vi "Torque_2.vi"() -> ()   [LabVIEW 2020]
uses:
  Support/Controls/Cmd_Mouse Popup.ctl
  Support/Controls/Clst_Initialize Input.ctl
  Support/Controls/Cmd_Var Data IO.ctl
  Variables/Global_Cal Info.vi
  Variables/Global_Constant.vi
panel:
  in  "타입":string
  in  "Measured CCW_ADJ":string[][](table) caption="● 조정후 지시값 (반시계방향)"
  in  "Measured CW_ADJ":string[][](table) caption="● 조정후 지시값 (시계방향)"
  in  "Measured CCW":string[][](table) caption="● 토크 교정기 지시값 (반시계방향)"
  in  "측정방향":enum16{"양방향", "시계방향", "반시계방향"}(ring)
  in  "Spec 변경":bool
  in  "Random":bool
  out "Spec":string[][](table) caption="Spec (N·m)"
  out "제목":string
  out "에러 출력":errorcluster
  out "Condition":string[][](table) caption="○ 토크렌치 정확도 교정"
  in  "최소눈금":string(combo)
  out "단위":string
  out "최대용량":string
  in  "Measured CW":string[][](table) caption="● 토크 교정기 지시값 (시계방향)"
  out "Load?":bool
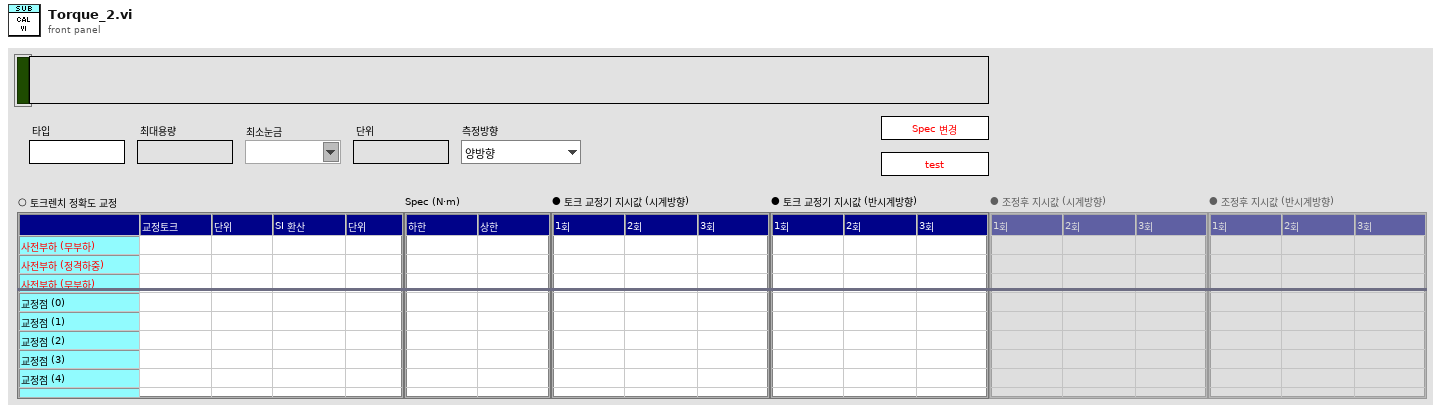
[diagram p1: front panel]
types:
  T1 = typedef "Clst_Cal Info Global.ctl" = cluster{"등록번호":string, "의뢰기관":string, "기기명":string, "제작회사":string, "형식":string, "기기번호":string, "소분류코드":string, "세부분류코드":string, "교정주기":string, "접수번호":string, "교정일자":string, "교정절차서 1":string, "교정절차서 2":string, "교정절차서 3":string, "접수확인자":string, "인증교정자":string, "기술책임자":string, "KOLAS 유무":string, "진행상태":string, "의뢰기관코드":string, "입고형태":string, "영문성적서?":bool, "합불판정?":bool, "부록?":bool, "절차서번호 1":string, "절차서번호 2":string, "절차서번호 3":string, "교정방식":string, "부서명":string}
  T2 = typedef "Cmd_Mouse Popup.ctl" = enum16{"활성화", "메뉴선택"}
  T3 = cluster{"Shift":bool, "Ctrl":bool, "Alt":bool, "Cmd":bool, "Opt":bool}
  T4 = typedef "Clst_Initialize Input.ctl" = cluster{"Initialize 1":cluster{"Condition":refnum<vi>[], "Spec":refnum<vi>[], "Measured":refnum<vi>[], "Resolution":refnum<vi>[], "Func_ext":string, "제목":refnum<vi>, "Measured_ADJ":refnum<vi>[]}, "Initialize 2":cluster{"문자열":refnum<vi>[], "콤보박스":refnum<vi>[], "링":refnum<vi>[], "열거형":refnum<vi>[], "테이블":refnum<vi>[], "여러열":refnum<vi>[], "디지털(DBL)":refnum<vi>[], "3D string":refnum<vi>[], "ctrl":refnum<vi>[], "boolean":refnum<vi>[]}}
  T5 = typedef "Cmd_Var Data IO.ctl" = enum16{"Condition", "Condition Default", "Condition_Temp", "Resolution", "Resolution Default", "Resolution Old", "Spec", "Spec Default", "Spec Old", "Spec Temp", "Result", "Result2", "Result3", "Result_Temp", "Result_ADJ", "Result_ADJ2", "STD1", "STD2", "STD3", "STD4", "STD5", "STD Temp", "CMC", "CMC Default"}
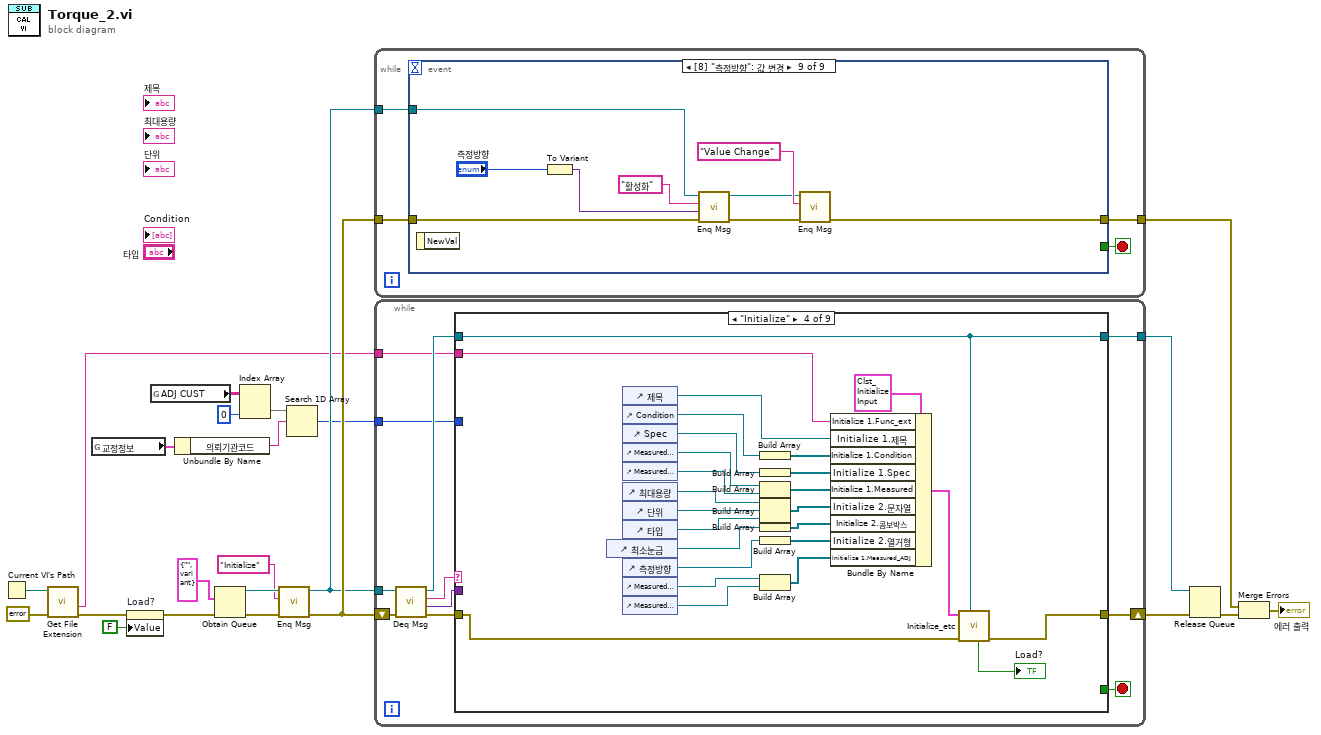
[diagram p0: block diagram]
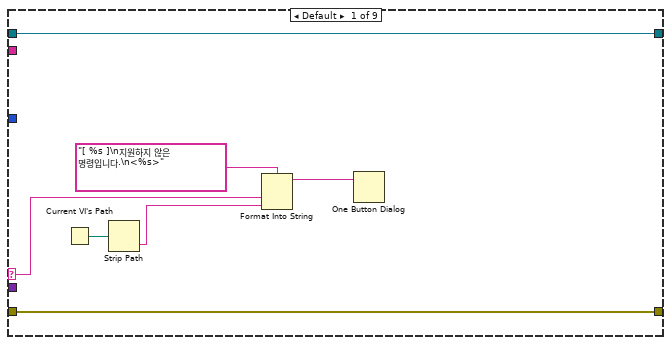
[diagram p2: hidden frame]
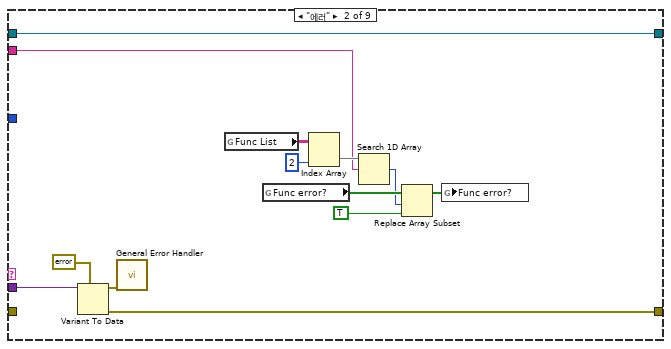
[diagram p3: hidden frame]
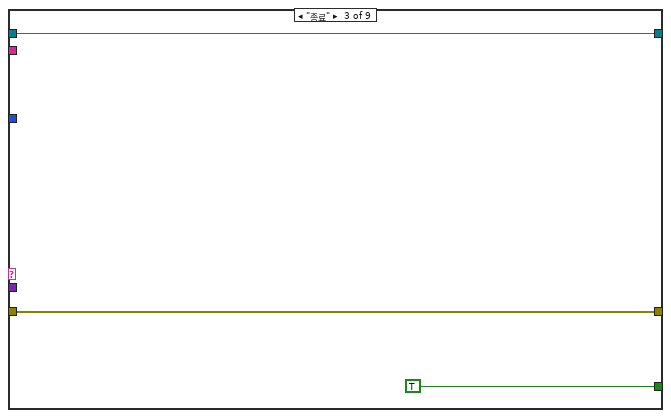
[diagram p4: hidden frame]
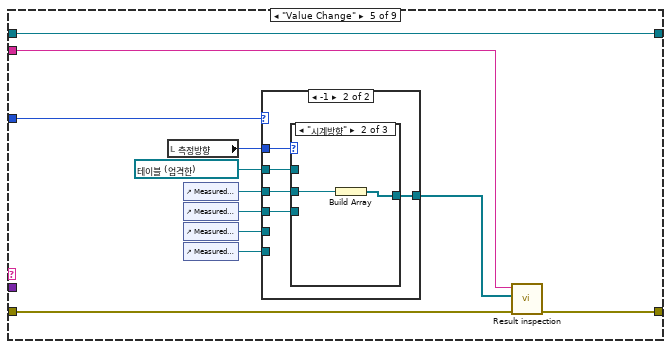
[diagram p5: hidden frame]
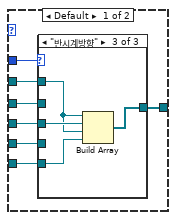
[diagram p6: hidden frame]
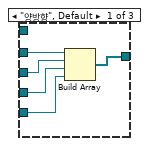
[diagram p7: hidden frame]
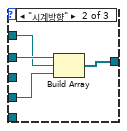
[diagram p8: hidden frame]
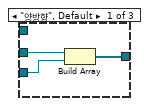
[diagram p9: hidden frame]
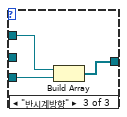
[diagram p10: hidden frame]
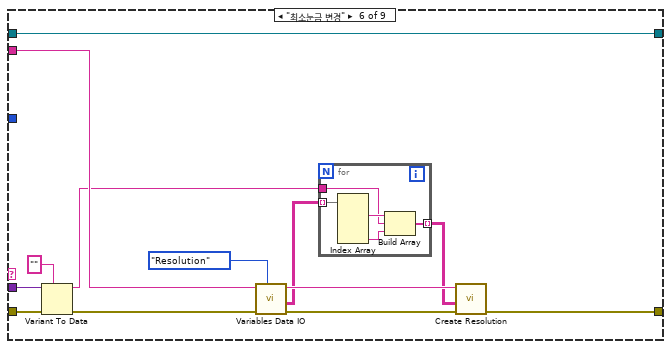
[diagram p11: hidden frame]
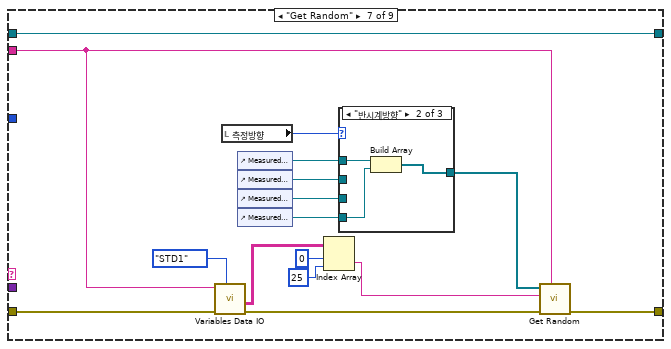
[diagram p12: hidden frame]
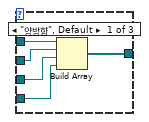
[diagram p13: hidden frame]
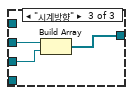
[diagram p14: hidden frame]
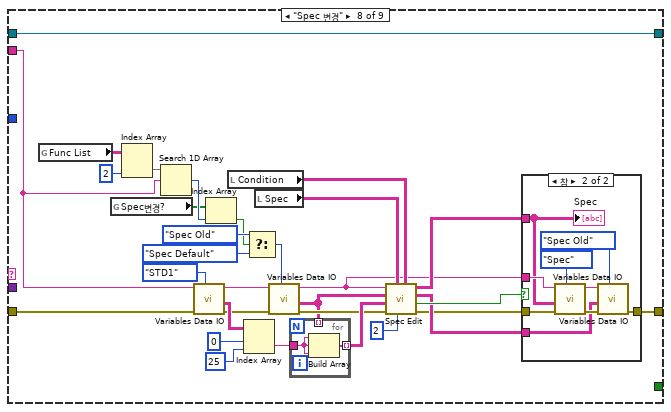
[diagram p15: hidden frame]
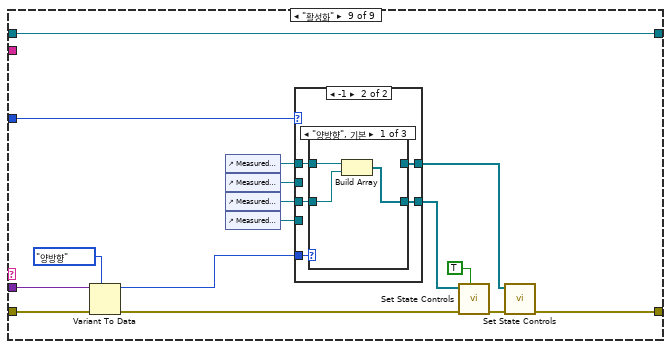
[diagram p17: hidden frame]
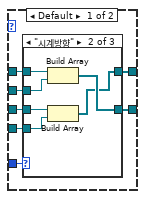
[diagram p18: hidden frame]
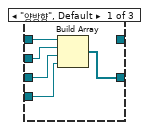
[diagram p19: hidden frame]
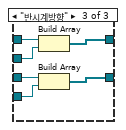
[diagram p20: hidden frame]
diagram:
  n1 = Current VI's Path() -> (path=w11:path)
  n2 = call <vilib>:"Get File Extension.vi"("error in (no error)"=errorcluster {"status"=FALSE, "code"=0, "source"=""} ("에러 상수"), "file"=w11) -> ("error out"=w2:errorcluster, "filename without extension"=w10:string)  [unwired: 5 in, 3 out]
  n3 = global read "Global_Cal Info.vi" "교정정보"() -> (w8:T1)
  n4 = property on="Load?" class="Bool (엄격한)"(error in=w2, "Value"=FALSE ("Load?")) -> (error out=w1:errorcluster)  [unwired: 1 in, 1 out]
  n5 = global read "Global_Constant.vi" "ADJ CUST"() -> (w7:string[][])
  n6 = Unbundle By Name(w8) -> ("의뢰기관코드"=w5:string)
  n7 = Obtain Queue(element data type=cluster{"메세지":string, "값":variant} {"메세지"="", "값"=variant} ("Message Cluster"), error in (no error)=w1) -> (queue out=w20:refnum<queue>, error out=w22:errorcluster)  [unwired: 3 in, 1 out]
  n8 = Index Array(array=w7, index (col)=0 ("비활성화된 인덱스 (열)")) -> (element=w6:string[])  [unwired: 1 in]
  n9 = call "Enq Msg.vi"("에러 입력(에러 없음)"=w22, "메세지"="Initialize", "큐 입력"=w20) -> ("에러 출력"=w21:errorcluster, "큐 출력"=w18:refnum<queue>)  [unwired: 7 in]
  n10 = Search 1D Array(1D array=w6, element=w5) -> (index of element=w4:i32)  [unwired: 1 in]
  n11 = while {
    tunnel: w21 -> [w25]
    tunnel: w18 -> [w26]
    tunnel: [w24] -> w15
    stop <- w27 stop-if-true
    n12 = event shown="[8] \"측정방향\": 값 변경" {
      selector: _ -> [_ _ _ _ _ _ _ _ _]
      dyn-events: _ -> [_ _ _ _ _ _ _ _ _]
      timeout: _ -> [_ _ _ _ _ _ _ _ _]
      tunnel: [w32 _ _ _ _ _ _ _ _] -> w27
      tunnel: w26 -> [w30 w37 w41 _ w48 _ w62 w68 w78]
      tunnel: w25 -> [w31 w38 w42 w45 w53 w60 w63 w70 w79]
      tunnel: [w28 w35 w39 w44 w47 w59 w61 w69 w73] -> w24
      event Panel Close? {
        w32 = TRUE ("버림?")
        n13 = event-data() -> ()  [unwired: 1 in, 1 out]
        n14 = call "Enq Msg.vi"("에러 입력(에러 없음)"=w31, "메세지"="종료", "큐 입력"=w30) -> ("에러 출력"=w28:errorcluster)  [unwired: 7 in, 1 out]
        n15 = event-data("Discard?"=w32) -> ()  [unwired: 1 in, 1 out]
      }
      event "최소눈금": Value Change {
        n16 = event-data() -> ()  [unwired: 1 in, 1 out]
        n17 = To Variant(anything="최소눈금") -> (Variant=w33:variant)
        n18 = call "Enq Msg.vi"("에러 입력(에러 없음)"=w38, "값"=w33, "메세지"="최소눈금 변경", "큐 입력"=w37) -> ("에러 출력"=w35:errorcluster)  [unwired: 6 in, 1 out]
      }
      event "Measured CW", "Measured CCW", "Measured CW_ADJ", "Measured CCW_ADJ": Value Change {
        n19 = event-data() -> ()  [unwired: 1 in, 1 out]
        n20 = call "Enq Msg.vi"("에러 입력(에러 없음)"=w42, "메세지"="Value Change", "큐 입력"=w41) -> ("에러 출력"=w39:errorcluster)  [unwired: 7 in, 1 out]
      }
      event "Condition", "Spec", "Measured CW", "Measured CCW", "Measured CW_ADJ", "Measured CCW_ADJ": Shortcut Menu Activation? {
        n21 = event-data() -> ("MenuRef"=w43:refnum<k9>)  [unwired: 1 in]
        n22 = call "Mouse PopUp Control.vi"("type"=Cmd_Mouse_Popup."활성화", "error in"=w45, "메뉴 참조"=w43) -> ("error out"=w44:errorcluster)  [unwired: 8 in]
        n23 = event-data() -> ()  [unwired: 2 in, 1 out]
      }
      event "Condition", "Spec", "Measured CW", "Measured CCW", "Measured CW_ADJ", "Measured CCW_ADJ": Shortcut Menu Selection (User) {
        n24 = event-data() -> ("CtlRef"=w51:refnum<vi>, "ItemTag"=w52:string)  [unwired: 1 in]
        n25 = call "Mouse PopUp Control.vi"("type"=Cmd_Mouse_Popup."메뉴선택", "error in"=w53, "아이템 태그"=w52, "Tbl 참조 번호"=w51) -> ("error out"=w49:errorcluster)  [unwired: 7 in]
        n26 = call "Enq Msg.vi"("에러 입력(에러 없음)"=w49, "메세지"="Value Change", "큐 입력"=w48) -> ("에러 출력"=w47:errorcluster)  [unwired: 7 in, 1 out]
      }
      event "Measured CW", "Measured CCW", "Condition", "Measured CW_ADJ", "Measured CCW_ADJ": Key Down; "Measured CW", "Measured CCW", "Condition", "Measured CW_ADJ", "Measured CCW_ADJ": Key Repeat {
        n27 = event-data() -> ("PlatMods"=w55:T3, "ScanCode"=w58:i16, "Mods.Num Pad"=w57:bool, "CtlRef"=w56:refnum<vi>)  [unwired: 1 in]
        n28 = call "Cursor Control.vi"("플랫폼 조합키"=w55, "참조"=w56, "Num Pad"=w57, "ScanCode"=w58, "error in"=w60) -> ("error out"=w59:errorcluster)  [unwired: 5 in, 1 out]
      }
      event "Random": Value Change {
        n29 = event-data() -> ()  [unwired: 1 in, 1 out]
        n30 = call "Enq Msg.vi"("에러 입력(에러 없음)"=w63, "메세지"="Get Random", "큐 입력"=w62) -> ("에러 출력"=w65:errorcluster, "큐 출력"=w66:refnum<queue>)  [unwired: 7 in]
        n31 = call "Enq Msg.vi"("에러 입력(에러 없음)"=w65, "메세지"="Value Change", "큐 입력"=w66) -> ("에러 출력"=w61:errorcluster)  [unwired: 7 in, 1 out]
      }
      event "Spec 변경": Value Change {
        n32 = event-data() -> ()  [unwired: 1 in, 1 out]
        n33 = call "Enq Msg.vi"("에러 입력(에러 없음)"=w70, "메세지"="Spec 변경", "큐 입력"=w68) -> ("에러 출력"=w69:errorcluster)  [unwired: 7 in, 1 out]
      }
      event "측정방향": Value Change {
        n34 = event-data() -> ()  [unwired: 1 in, 1 out]
        n35 = To Variant(anything="측정방향") -> (Variant=w77:variant)
        n36 = call "Enq Msg.vi"("에러 입력(에러 없음)"=w79, "값"=w77, "메세지"="활성화", "큐 입력"=w78) -> ("에러 출력"=w74:errorcluster, "큐 출력"=w72:refnum<queue>)  [unwired: 6 in]
        n37 = call "Enq Msg.vi"("에러 입력(에러 없음)"=w74, "메세지"="Value Change", "큐 입력"=w72) -> ("에러 출력"=w73:errorcluster)  [unwired: 7 in, 1 out]
      }
    }
  }
  n38 = while {
    shift-right: [w91] -> w17
    shift-left: w21 -> [w90]
    tunnel: w18 -> [w88]
    tunnel: [w83] -> w16
    tunnel: w10 -> [w82]
    tunnel: w4 -> [w81]
    stop <- w84 stop-if-true
    n39 = call "Deq Msg.vi"("에러 입력(에러 없음)"=w90, "큐 입력"=w88) -> ("에러 출력"=w89:errorcluster, "값"=w85:variant, "메세지"=w87:string, "큐 출력"=w86:refnum<queue>)  [unwired: 6 in]
    n40 = case shown="\"Initialize\"" w87 {
      selector: w87 -> [w94 _ _ _ _ _ _ _ _]
      tunnel: w89 -> [w98 _ w114 w116 w147 w197 w213 w233 w288]
      tunnel: [w98 w108 w114 w126 w151 w189 w217 w234 w278] -> w91
      tunnel: w86 -> [w97 w107 w112 w127 w152 w198 w219 w261 w289]
      tunnel: w85 -> [_ w109 _ _ _ w196 _ _ w287]
      tunnel: [_ _ TRUE ("버림?") _ _ _ _ _ _] -> w84
      tunnel: [w97 w107 w112 w127 w152 w198 w219 w261 w289] -> w83
      tunnel: w82 -> [_ w99 _ w128 w150 w191 w214 w232 _]
      tunnel: w81 -> [_ _ _ _ w141 _ _ _ w274]
      frame Default {
        n41 = Current VI's Path() -> (path=w93:path)
        n42 = Strip Path(path=w93) -> (name=w92:string)  [unwired: 1 out]
        n43 = Format Into String(format string="[ %s ]\n지원하지 않은 명령입니다.\n<%s>" ("메시지"), w94, w92) -> (resulting string=w95:string)  [unwired: 2 in, 1 out]
        n44 = One Button Dialog(message=w95) -> ()  [unwired: 1 in, 1 out]
      }
      frame "에러" {
        n45 = Variant To Data(type=errorcluster {"status"=FALSE, "code"=0, "source"=""} ("에러 출력"), Variant=w109) -> (data=w111:errorcluster, error out=w108:errorcluster)  [unwired: 1 in]
        n46 = call <vilib>:"General Error Handler.vi"("error in (no error)"=w111) -> ()  [unwired: 10 in, 5 out]
        n47 = global read "Global_Cal Info.vi" "Func List"() -> (w105:string[][])
        n48 = global read "Global_Cal Info.vi" "Func error?"() -> (w102:bool[])
        n49 = Index Array(array=w105, index (col)=2 ("비활성화된 인덱스 (열)")) -> (element=w104:string[])  [unwired: 1 in]
        n50 = Search 1D Array(1D array=w104, element=w99) -> (index of element=w101:i32)  [unwired: 1 in]
        n51 = Replace Array Subset(array=w102, new element=TRUE ("새 원소/부분배열"), index=w101) -> (w100:bool[])
        n52 = global write "Global_Cal Info.vi" "Func error?"(w100) -> ()
      }
      frame "종료" {
      }
      frame "Initialize" {
        n53 = control-ref of="최소눈금"() -> (w134:refnum<vi>)
        n54 = control-ref of="제목"() -> (w132:refnum<vi>)
        n55 = control-ref of="Condition"() -> (w125:refnum<vi>)
        n56 = control-ref of="Spec"() -> (w121:refnum<vi>)
        n57 = control-ref of="Measured CW"() -> (w136:refnum<vi>)
        n58 = control-ref of="Measured CCW"() -> (w124:refnum<vi>)
        n59 = control-ref of="최대용량"() -> (w131:refnum<vi>)
        n60 = control-ref of="단위"() -> (w130:refnum<vi>)
        n61 = control-ref of="타입"() -> (w115:refnum<vi>)
        n62 = control-ref of="측정방향"() -> (w122:refnum<vi>)
        n63 = control-ref of="Measured CW_ADJ"() -> (w119:refnum<vi>)
        n64 = control-ref of="Measured CCW_ADJ"() -> (w120:refnum<vi>)
        n65 = Build Array(w125) -> (w138:refnum<vi>[])
        n66 = Build Array(w121) -> (w129:refnum<vi>[])
        n67 = Build Array(w136, w124) -> (w137:refnum<vi>[])
        n68 = Build Array(w131, w130, w115) -> (w135:refnum<vi>[])
        n69 = Build Array(w134) -> (w133:refnum<vi>[])
        n70 = Build Array(w122) -> (w123:refnum<vi>[])
        n71 = Build Array(w119, w120) -> (w118:refnum<vi>[])
        n72 = Bundle By Name(cluster=T4 {"Initialize 1"={"Condition"=[], "Spec"=[], "Measured"=[], "Resolution"=[], "Func_ext"="", "제목"=refnum, "Measured_ADJ"=[]}, "Initialize 2"={"문자열"=[], "콤보박스"=[], "링"=[], "열거형"=[], "테이블"=[], "여러열"=[], "디지털(DBL)"=[], "3D string"=[], "ctrl"=[], "boolean"=[]}} ("입력 클러스터"), "Initialize 1.Func_ext"=w128, "Initialize 1.제목"=w132, "Initialize 1.Condition"=w138, "Initialize 1.Spec"=w129, "Initialize 1.Measured"=w137, "Initialize 2.문자열"=w135, "Initialize 2.콤보박스"=w133, "Initialize 2.열거형"=w123, "Initialize 1.Measured_ADJ"=w118) -> (w139:T4)
        n73 = call "Initialize_etc.vi"("큐 입력"=w127, "error in"=w116, "입력 클러스터"=w139) -> ("error out"=w126:errorcluster, "Load?"=→"Load?":bool)  [unwired: 6 in, 1 out]
      }
      frame "Value Change" {
        n74 = local read "측정방향"() -> (w145:enum16{"양방향", "시계방향", "반시계방향"})
        n75 = control-ref of="Measured CW"() -> (w149:refnum<vi>)
        n76 = control-ref of="Measured CCW"() -> (w146:refnum<vi>)
        n77 = control-ref of="Measured CW_ADJ"() -> (w143:refnum<vi>)
        n78 = control-ref of="Measured CCW_ADJ"() -> (w142:refnum<vi>)
        n79 = case shown="-1" w141 {
          tunnel: w149 -> [w159 w177]
          tunnel: [w158 w176] -> w148
          tunnel: w146 -> [w157 w175]
          tunnel: w145 -> [w156 w174]
          tunnel: refnum<vi> refnum ("Measured CW") -> [w155 w173]
          tunnel: w143 -> [w154 _]
          tunnel: w142 -> [w153 _]
          frame Default {
            n80 = case shown="\"반시계방향\"" w156 {
              tunnel: w159 -> [w164 w168 _]
              tunnel: [w163 w167 w172] -> w158
              tunnel: w157 -> [w162 _ w170]
              tunnel: w155 -> [_ w166 w169]
              tunnel: w154 -> [w161 w165 _]
              tunnel: w153 -> [w160 _ w171]
              frame "양방향", Default {
                n81 = Build Array(w164, w162, w161, w160) -> (w163:refnum<vi>[])
              }
              frame "시계방향" {
                n82 = Build Array(w168, w166, w165) -> (w167:refnum<vi>[])
              }
              frame "반시계방향" {
                n83 = Build Array(w169, w170, w169, w171) -> (w172:refnum<vi>[])
              }
            }
          }
          frame -1 {
            n84 = case shown="\"시계방향\"" w174 {
              tunnel: w177 -> [w180 w182 _]
              tunnel: [w179 w181 w185] -> w176
              tunnel: w175 -> [w178 _ w184]
              tunnel: w173 -> [_ _ w183]
              frame "양방향", Default {
                n85 = Build Array(w180, w178) -> (w179:refnum<vi>[])
              }
              frame "시계방향" {
                n86 = Build Array(w182) -> (w181:refnum<vi>[])
              }
              frame "반시계방향" {
                n87 = Build Array(w183, w184) -> (w185:refnum<vi>[])
              }
            }
          }
        }
        n88 = call "Result inspection.vi"("error in"=w147, "Ref. Data (Inspection)"=w148, "Func ext"=w150) -> ("error out"=w151:errorcluster)  [unwired: 5 in, 3 out]
      }
      frame "최소눈금 변경" {
        n89 = Variant To Data(error in=w197, type="", Variant=w196) -> (data=w188:string, error out=w190:errorcluster)
        n90 = call "Variables Data IO.vi"("Select"=Cmd_Var_Data_IO."Resolution", "error in"=w190, "Func_ext"=w191) -> ("error out"=w193:errorcluster, "Data Out"=w187:string[][], "Func_ext Out"=w192:string)  [unwired: 6 in]
        n91 = for {
          tunnel: w187 -> [w203] mode=indexing
          tunnel: w188 -> [w201]
          tunnel: [w199] -> w186 mode=indexing
          n92 = Index Array(array=w203) -> (element #1=w202:string, element #4=w200:string)  [unwired: 4 in, 2 out]
          n93 = Build Array(w202, w201, w200) -> (w199:string[])
        }
        n94 = call "Create Resolution.vi"("에러 입력(에러 없음)"=w193, "Resolution"=w186, "Func_ext"=w192) -> ("에러 출력"=w189:errorcluster)  [unwired: 6 in, 2 out]
      }
      frame "Get Random" {
        n95 = call "Variables Data IO.vi"("Select"=Cmd_Var_Data_IO."STD1", "error in"=w213, "Func_ext"=w214) -> ("error out"=w212:errorcluster, "Data Out"=w210:string[][])  [unwired: 6 in, 1 out]
        n96 = local read "측정방향"() -> (w206:enum16{"양방향", "시계방향", "반시계방향"})
        n97 = control-ref of="Measured CCW"() -> (w216:refnum<vi>)
        n98 = control-ref of="Measured CW"() -> (w215:refnum<vi>)
        n99 = control-ref of="Measured CW_ADJ"() -> (w205:refnum<vi>)
        n100 = control-ref of="Measured CCW_ADJ"() -> (w204:refnum<vi>)
        n101 = Index Array(array=w210, index (row)=0 ("인덱스 (행)"), index (col)=25 ("비활성화된 인덱스 (열)")) -> (element=w207:string)
        n102 = case shown="\"반시계방향\"" w206 {
          tunnel: [w224 w227 w230] -> w218
          tunnel: w216 -> [w223 w226 _]
          tunnel: w215 -> [w222 _ w229]
          tunnel: w205 -> [w221 _ w228]
          tunnel: w204 -> [w220 w225 _]
          frame "양방향", Default {
            n103 = Build Array(w223, w222, w221, w220) -> (w224:refnum<vi>[])
          }
          frame "반시계방향" {
            n104 = Build Array(w226, w225) -> (w227:refnum<vi>[])
          }
          frame "시계방향" {
            n105 = Build Array(w229, w228) -> (w230:refnum<vi>[])
          }
        }
        n106 = call "Get Random.vi"("Func_Ext"=w214, "에러 입력"=w212, "분해능"=w207, "Meas"=w218) -> ("에러 출력"=w217:errorcluster)  [unwired: 6 in, 1 out]
      }
      frame "Spec 변경" {
        n107 = global read "Global_Cal Info.vi" "Func List"() -> (w240:string[][])
        n108 = global read "Global_Cal Info.vi" "Spec변경?"() -> (w236:bool[])
        n109 = Index Array(array=w240, index (col)=2 ("비활성화된 인덱스 (열)")) -> (element=w238:string[])  [unwired: 1 in]
        n110 = Search 1D Array(1D array=w238, element=w232) -> (index of element=w237:i32)  [unwired: 1 in]
        n111 = call "Variables Data IO.vi"("Select"=Cmd_Var_Data_IO."STD1", "error in"=w233, "Func_ext"=w232) -> ("error out"=w247:errorcluster, "Data Out"=w250:string[][], "Func_ext Out"=w246:string)  [unwired: 6 in]
        n112 = Index Array(array=w236, index=w237) -> (element=w241:bool)
        n113 = local read "Condition"() -> (w255:string[][])
        n114 = Index Array(array=w250, index (row)=0 ("비활성화된 인덱스 (행)"), index (col)=25 ("인덱스 (행)")) -> (element=w253:string)
        n115 = Select(t=Cmd_Var_Data_IO."Spec Old" ("Select"), s=w241, f=Cmd_Var_Data_IO."Spec Default" ("Select")) -> (s? t:f=w235:T5)
        n116 = local read "Spec"() -> (w256:string[][])
        n117 = call "Variables Data IO.vi"("Select"=w235, "error in"=w247, "Func_ext"=w246) -> ("error out"=w245:errorcluster, "Data Out"=w231:string[][], "Func_ext Out"=w251:string)  [unwired: 6 in]
        n118 = for {
          tunnel: [w262] -> w254 mode=indexing
          tunnel: w253 -> [w263]
          tunnel: w231 -> [_] mode=indexing
          n119 = Build Array(w263, w263, w263) -> (w262:string[])
        }
        n120 = call "Spec Edit.vi"("Condition"=w255, "열번호(기준값)"=2 ("기준열(0)"), "Spec Value"=w256, "에러 입력(에러 없음)"=w245, "Resolution"=w254, "Spec Default"=w231, "Func_ext"=w251) -> ("에러 출력"=w252:errorcluster, "변경?"=w260:bool, "Spec Default out"=w259:string[][], "Spec 출력"=w257:string[][])  [unwired: 1 in]
        n121 = case shown="참" w260 {
          tunnel: w252 -> [w264 w272]
          tunnel: [w264 w269] -> w234
          tunnel: w257 -> [_ w265]
          tunnel: w251 -> [_ w271]
          tunnel: w259 -> [_ w266]
          frame False {
          }
          frame True {
            n122 = call "Variables Data IO.vi"("Select"=Cmd_Var_Data_IO."Spec", "error in"=w272, "Data In"=w265, "Func_ext"=w271) -> ("error out"=w270:errorcluster, "Func_ext Out"=w267:string)  [unwired: 5 in, 1 out]
            n123 = call "Variables Data IO.vi"("Select"=Cmd_Var_Data_IO."Spec Old", "error in"=w270, "Data In"=w266, "Func_ext"=w267) -> ("error out"=w269:errorcluster)  [unwired: 5 in, 2 out]
            "Spec" <- w265
          }
        }
      }
      frame "활성화" {
        n124 = Variant To Data(error in=w288, type=enum16{"양방향", "시계방향", "반시계방향"}."양방향" ("측정방향 2"), Variant=w287) -> (data=w284:enum16{"양방향", "시계방향", "반시계방향"}, error out=w285:errorcluster)
        n125 = control-ref of="Measured CW"() -> (w283:refnum<vi>)
        n126 = control-ref of="Measured CW_ADJ"() -> (w276:refnum<vi>)
        n127 = control-ref of="Measured CCW"() -> (w282:refnum<vi>)
        n128 = control-ref of="Measured CCW_ADJ"() -> (w275:refnum<vi>)
        n129 = case shown="-1" w274 {
          tunnel: w284 -> [w296 w318]
          tunnel: w283 -> [w295 w317]
          tunnel: w282 -> [w294 w316]
          tunnel: [w293 w315] -> w281
          tunnel: [w292 w314] -> w277
          tunnel: w276 -> [w291 _]
          tunnel: w275 -> [w290 _]
          frame Default {
            n130 = case shown="\"시계방향\"" w296 {
              tunnel: w295 -> [w301 w307 w313]
              tunnel: w294 -> [w300 w305 w312]
              tunnel: [w299 w306 w311] -> w293
              tunnel: [_ w304 w310] -> w292
              tunnel: w291 -> [w298 w303 w309]
              tunnel: w290 -> [w297 w302 w308]
              frame "양방향", Default {
                n131 = Build Array(w301, w298, w300, w297) -> (w299:refnum<vi>[])
              }
              frame "시계방향" {
                n132 = Build Array(w307, w303) -> (w306:refnum<vi>[])
                n133 = Build Array(w305, w302) -> (w304:refnum<vi>[])
              }
              frame "반시계방향" {
                n134 = Build Array(w313, w309) -> (w310:refnum<vi>[])
                n135 = Build Array(w312, w308) -> (w311:refnum<vi>[])
              }
            }
          }
          frame -1 {
            n136 = case shown="\"양방향\", 기본" w318 {
              tunnel: w317 -> [w321 w325 w329]
              tunnel: w316 -> [w320 w323 w328]
              tunnel: [w319 w324 w327] -> w315
              tunnel: [_ w322 w326] -> w314
              frame "양방향", Default {
                n137 = Build Array(w321, w320) -> (w319:refnum<vi>[])
              }
              frame "시계방향" {
                n138 = Build Array(w325) -> (w324:refnum<vi>[])
                n139 = Build Array(w323) -> (w322:refnum<vi>[])
              }
              frame "반시계방향" {
                n140 = Build Array(w329) -> (w326:refnum<vi>[])
                n141 = Build Array(w328) -> (w327:refnum<vi>[])
              }
            }
          }
        }
        n142 = call "Set State Controls.vi"("활성화 (F)"=TRUE, "error in (no error)"=w285, "컨트롤 참조 배열 in"=w281) -> ("error out"=w279:errorcluster)  [unwired: 7 in, 1 out]
        n143 = call "Set State Controls.vi"("error in (no error)"=w279, "컨트롤 참조 배열 in"=w277) -> ("error out"=w278:errorcluster)  [unwired: 8 in, 1 out]
      }
    }
  }
  n144 = Release Queue(queue=w16, error in (no error)=w17) -> (error out=w14:errorcluster)  [unwired: 1 in, 2 out]
  n145 = Merge Errors(w15, w14) -> (→"에러 출력":errorcluster)
